vi "Encoder Position & Velocity (FPGA).vi"(3 "Velocity Interval (uSec)":u32=1000, 5 "Position Reset":bool) -> (0 "Velocity (Counts/Interval)":i32, 1 "Acceleration (Counts/Interval)":i32, 2 "Position (Counts)":i32)   [LabVIEW 2013]
doc: "This is an FPGA vi for Quadrature Encoder Velocity and Acceleration Estimation using CompactRIO. It requires as inputs a Fixed Time Interval for velocity and acceleration estimation.\n\nThis application is designed to work with an R-Series expansion setup using PCI/PXI-7811R FPGA device and a CompactRIO cRIO-9411 digital input module installed in slot 1 of the expansion chassis."
uses:
  <vilib>/rvi/Emulation/niFpgaSctlEmulationGetInTimedLoop.vi
  <vilib>/rvi/Emulation/niFpgaEmulationReportErrorSimple.vi
  <vilib>/rvi/Emulation/niFpgaGetClockAttributes.vi
  <vilib>/rvi/eio/common/nirviEmuTemplateMethod_errors.vi
  <vilib>/rvi/Emulation/niFpgaCriticalErrorInLSC.vi
  <vilib>/rvi/Arithmetic/AddSubMult/XNode/nirviSatArithmetic.xnode
  <vilib>/eio/EIONode/EIONode.xnode
panel:
  in  "stop":bool
  # "FPGA Application for Quadrature Encoder Velocity and \nAcceleration Estimation using CompactRIO.\n\nThis application is designed to work with an R-Series expansion setup \nusing FPGA-7811R and a CompactRIO cRIO-9411 digital input module \ninstalled in slot 1 of the expansion chassis."
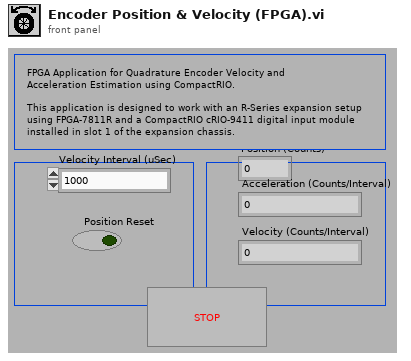
[diagram p1: front panel]
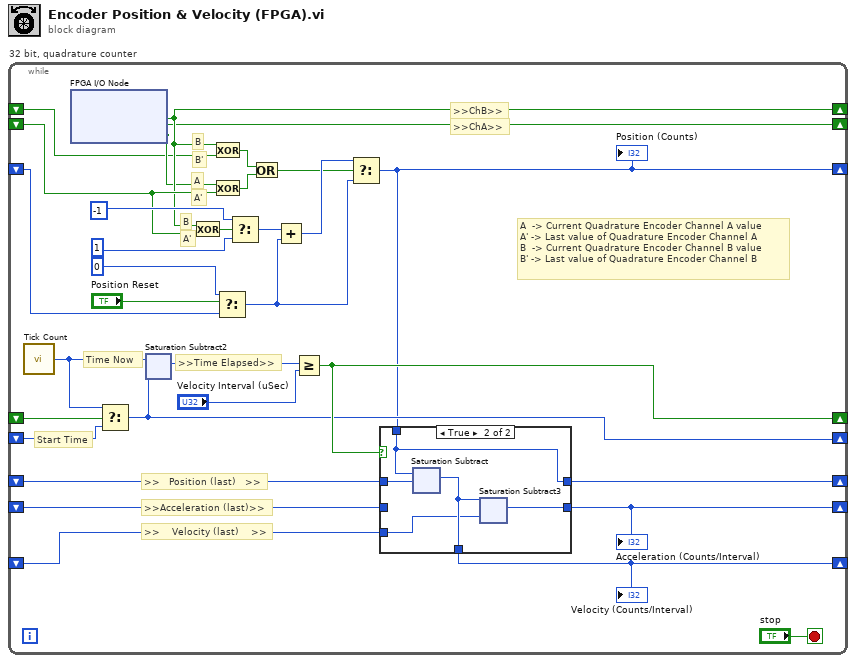
[diagram p0: block diagram]
diagram:
  n1 = while "32 bit, quadrature counter" {
    shift-right: [w20] -> _
    shift-left: _ -> [w5]
    shift-right: [w4] -> _
    shift-left: _ -> [w16]
    shift-right: [w19] -> _
    shift-left: _ -> [w21]
    shift-right: [w12] -> _
    shift-left: _ -> [w15]
    shift-right: [w7] -> _
    shift-left: _ -> [w13]
    shift-right: [w1] -> _
    shift-left: _ -> [w10]
    shift-right: [w2] -> _
    shift-left: _ -> [w9]
    shift-right: [w3] -> _
    shift-left: _ -> [w6]
    stop <- "stop" stop-if-true
    # "A  -> Current Quadrature Encoder Channel A value\nA' -> Last value of Quadrature Encoder Channel A\nB  -> Current Quadrature Encoder Channel B value\nB' -> Last value of Quadrature Encoder Channel B"
    # ">>Acceleration (last)>>"
    # "Start Time"
    # "A'"
    # "B"
    # "A'"
    # "A"
    # "B'"
    # "B"
    # ">>ChB>>"
    # ">>ChA>>"
    # ">>    Velocity (last)    >>"
    # ">>   Position (last)   >>"
    # "Time Now"
    # ">>Time Elapsed>>"
    n2 = call "Tick Count"() -> ("Tick Count(uSec)"=w8:u32)
    n3 = xnode "FPGA I/O Node"() -> ("Mod1/DI2"=w20:bool, "Mod1/DI0"=w19:bool)  [unwired: 2 in, 2 out]
    n4 = Select(t=w8, s=w15, f=w13) -> (s? t:f=w7:u32)
    n5 = xnode ("Saturation Subtract2")("x"=w8, "y"=w7) -> ("x-y"=w11:u32)
    n6 = Exclusive Or(1:w21, 2:w20) -> (0:w22:bool)
    n7 = Exclusive Or(1:w5, 2:w20) -> (0:w23:bool)
    n8 = Exclusive Or(1:w21, 2:w19) -> (0:w24:bool)
    n9 = Select(t=0 ("32 bit"), s="Position Reset", f=w16) -> (s? t:f=w29:i32)
    n10 = Select(t=-1 ("32 bit"), s=w22, f=1 ("32 bit")) -> (s? t:f=w27:i32)
    n11 = Or(x=w23, y=w24) -> (x .or. y?=w17:bool)
    n12 = Add(x=w27, y=w29) -> (x+y=w31:i32)
    n13 = Greater Or Equal?(x=w11, y="Velocity Interval (uSec)") -> (x >= y?=w12:bool)
    n14 = Select(t=w31, s=w17, f=w29) -> (s? t:f=w4:i32)
    "Position (Counts)" <- w4
    n15 = case shown="True" w12 {
      tunnel: w4 -> [_ w45]
      tunnel: w10 -> [w42 w49]
      tunnel: [w44 w48] -> w2
      tunnel: w9 -> [w44 w47]
      tunnel: [w43 w46] -> w3
      tunnel: w6 -> [w43 _]
      tunnel: [w42 w45] -> w1
      frame False {
      }
      frame True {
        n16 = xnode ("Saturation Subtract")("x"=w45, "y"=w49) -> ("x-y"=w48:i32)
        n17 = xnode ("Saturation Subtract3")("x"=w48, "y"=w47) -> ("x-y"=w46:i32)
      }
    }
    "Acceleration (Counts/Interval)" <- w3
    "Velocity (Counts/Interval)" <- w2
  }
